vi "readMotorPodTurret.vi"(7 "Input Pod Clustor":T1, 8 "Pod Number":i32, 9 "Refnum in":T2) -> (1 "output cluster":T1)   [LabVIEW 2014]
uses:
  <vilib>/Utility/config.llb/Config Data RefNum.ctl
  read/readBooleanKey.vi
  read/readDoubleKey.vi
  read/readI32.vi
  read/readStringKey.vi
  <vilib>/Utility/config.llb/NI_LVConfig.lvlib
panel:
  in  "error in (no error)":errorcluster
  out "Refnum out":T2
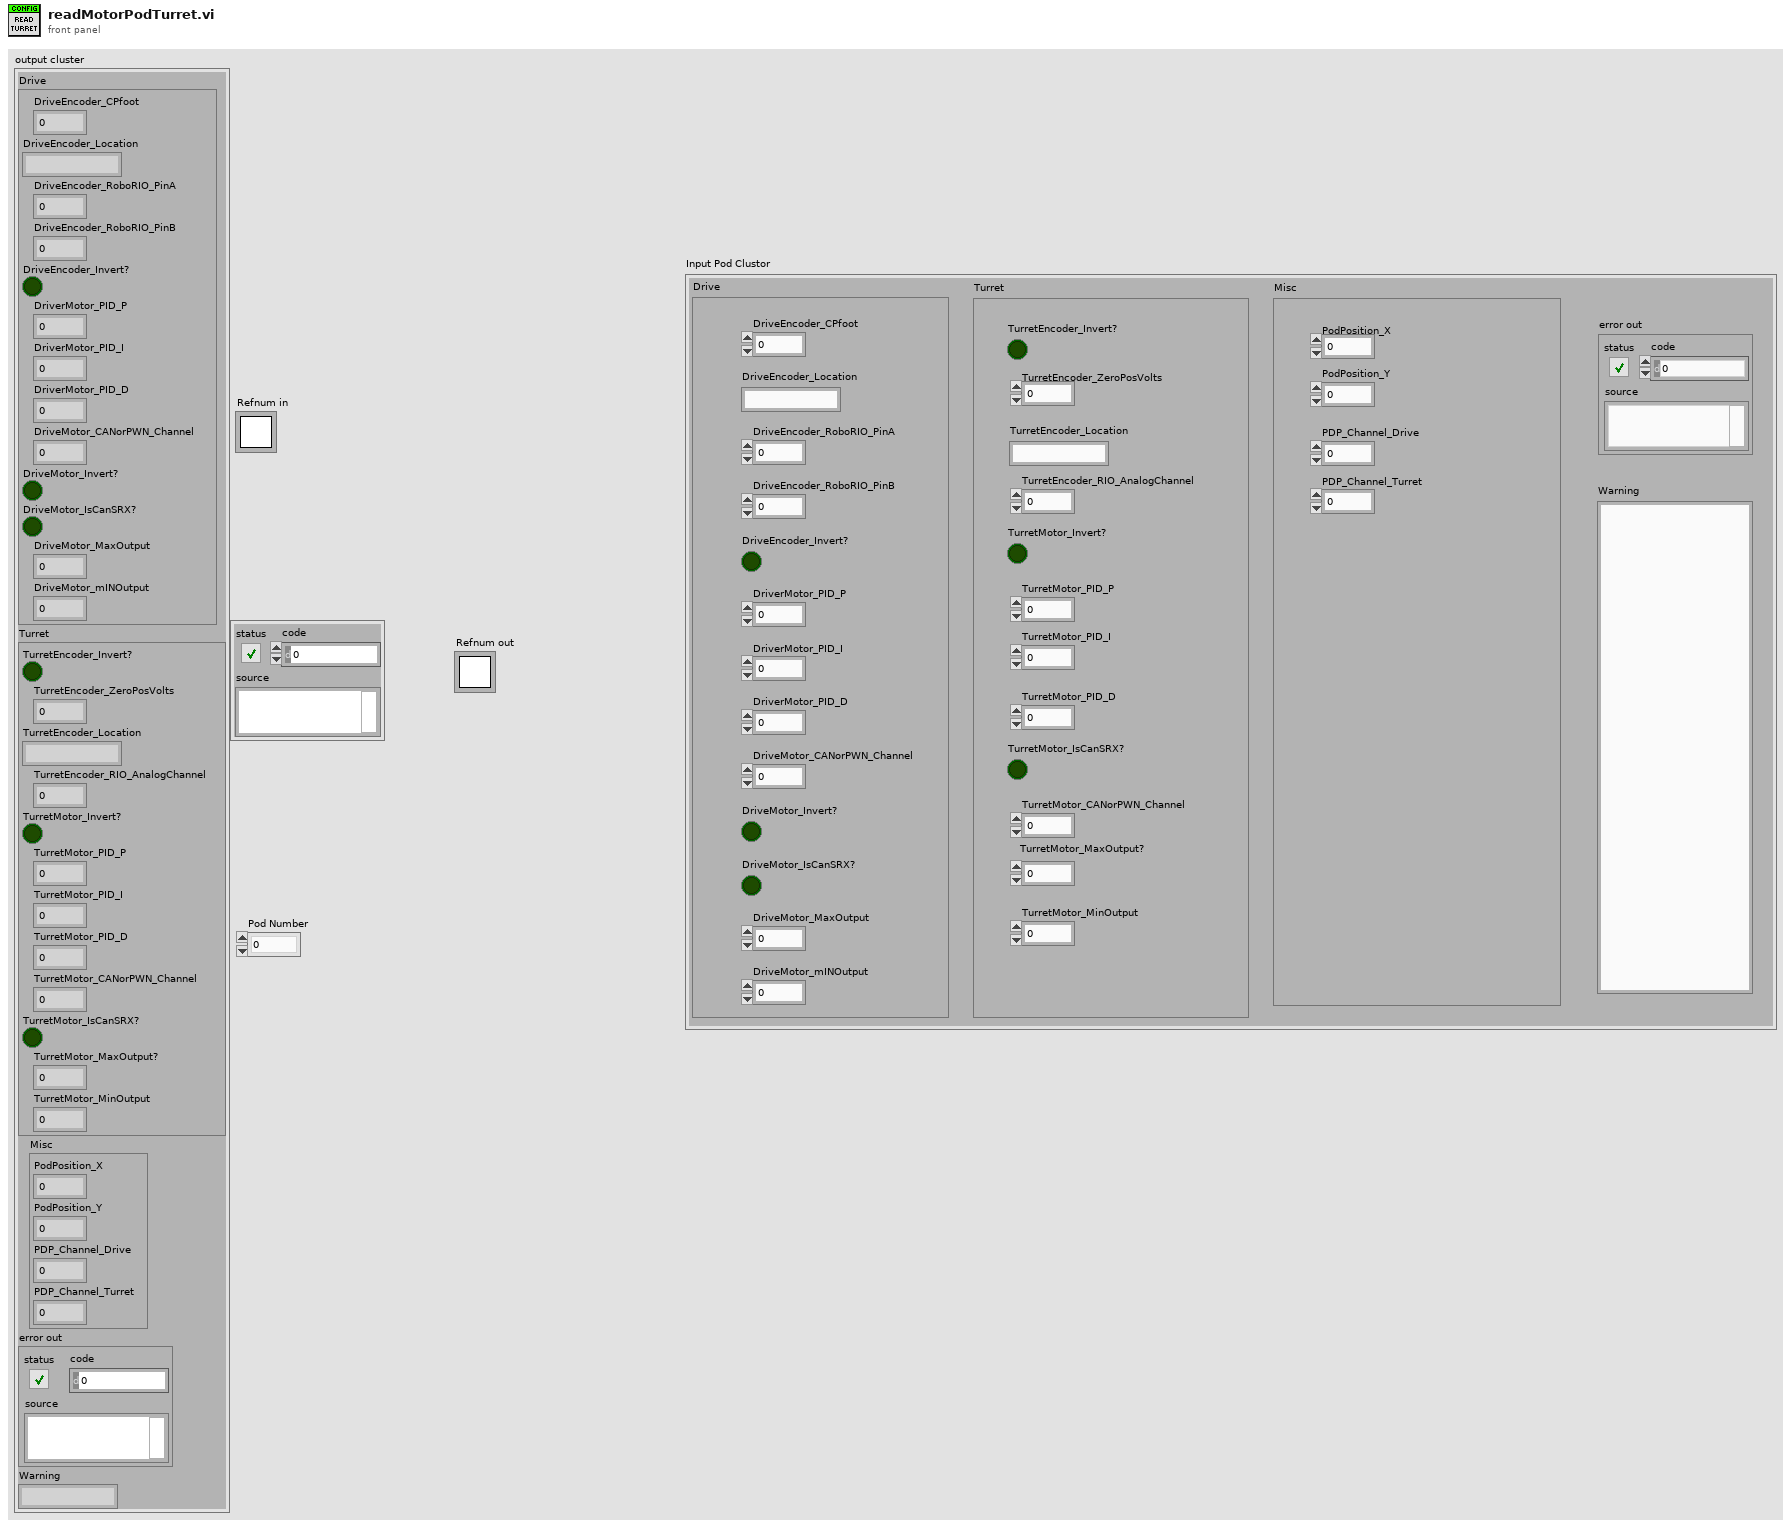
[diagram p1: front panel]
types:
  T1 = cluster{"Drive":cluster{"DriveEncoder_CPfoot":dbl, "DriveEncoder_Location":string, "DriveEncoder_RoboRIO_PinA":i32, "DriveEncoder_RoboRIO_PinB":i32, "DriveEncoder_Invert?":bool, "DriverMotor_PID_P":dbl, "DriverMotor_PID_I":dbl, "DriverMotor_PID_D":dbl, "DriveMotor_CANorPWN_Channel":i32, "DriveMotor_Invert?":bool, "DriveMotor_IsCanSRX?":bool, "DriveMotor_MaxOutput":dbl, "DriveMotor_mINOutput":dbl}, "Turret":cluster{"TurretEncoder_Invert?":bool, "TurretEncoder_ZeroPosVolts":dbl, "TurretEncoder_Location":string, "TurretEncoder_RIO_AnalogChannel":dbl, "TurretMotor_Invert?":bool, "TurretMotor_PID_P":dbl, "TurretMotor_PID_I":dbl, "TurretMotor_PID_D":dbl, "TurretMotor_CANorPWN_Channel":dbl, "TurretMotor_IsCanSRX?":bool, "TurretMotor_MaxOutput?":dbl, "TurretMotor_MinOutput":dbl}, "Misc":cluster{"PodPosition_X":dbl, "PodPosition_Y":dbl, "PDP_Channel_Drive":i32, "PDP_Channel_Turret":i32}, "error out":errorcluster, "Warning":string}
  T2 = typedef "NI_LVConfig.lvlib/Config Data RefNum.ctl" = refnum<k1>
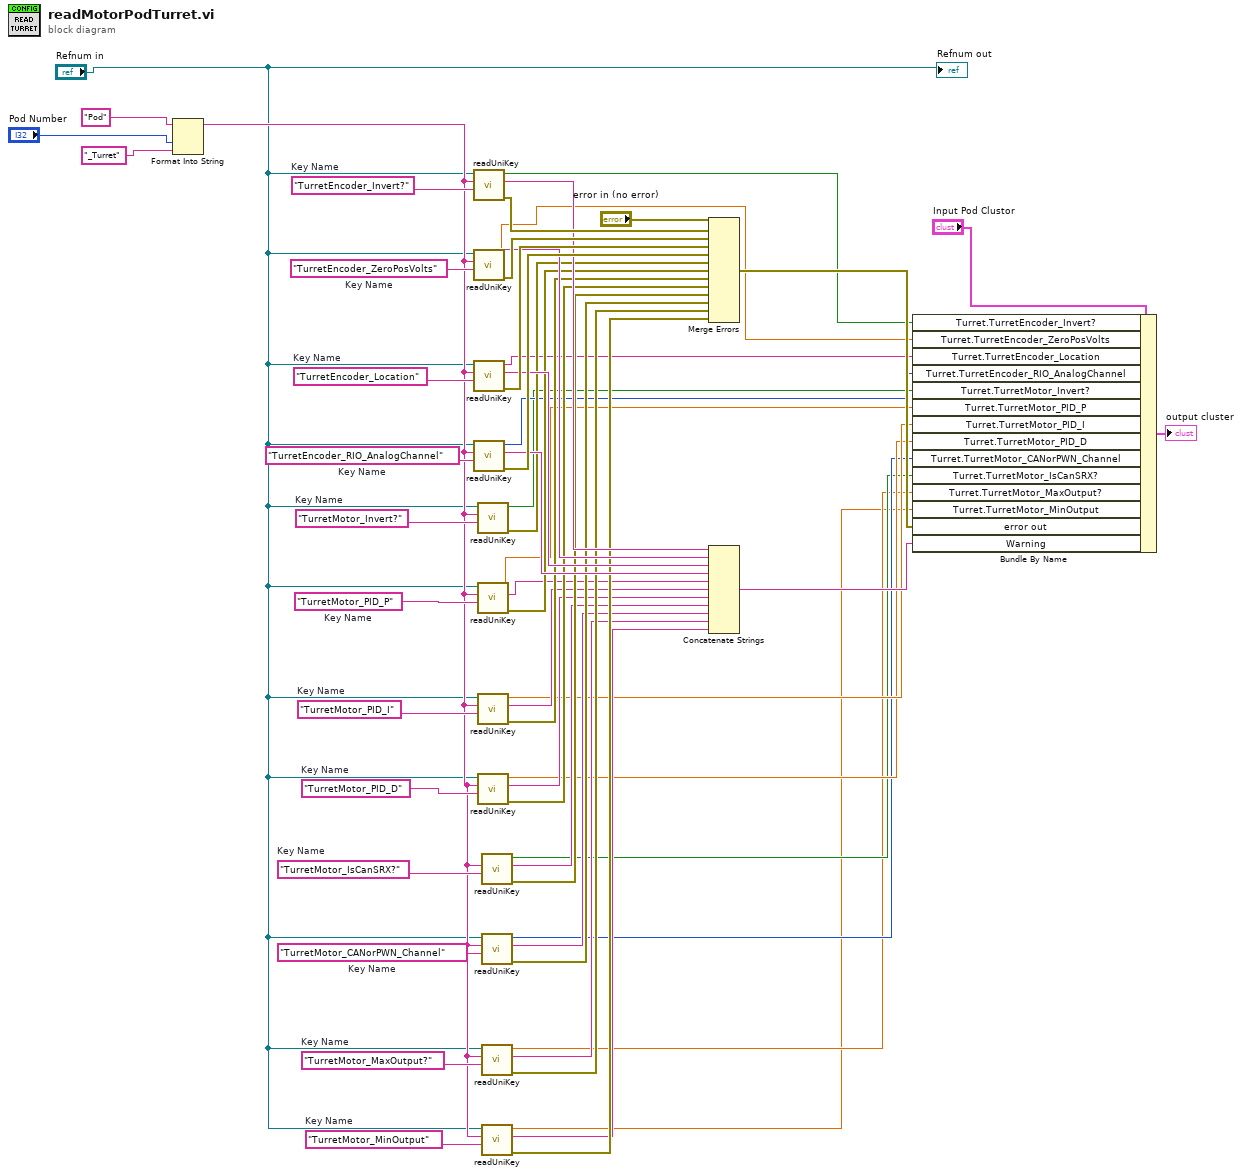
[diagram p0: block diagram]
diagram:
  w36 = "TurretMotor_MinOutput"  # Key Name
  w35 = "TurretMotor_MaxOutput?"  # Key Name
  w37 = "TurretMotor_CANorPWN_Channel"  # Key Name
  w38 = "TurretMotor_IsCanSRX?"  # Key Name
  w41 = "TurretMotor_PID_D"  # Key Name
  w42 = "TurretMotor_PID_I"  # Key Name
  w40 = "TurretMotor_PID_P"  # Key Name
  w39 = "TurretMotor_Invert?"  # Key Name
  w55 = "TurretEncoder_RIO_AnalogChannel"  # Key Name
  w54 = "TurretEncoder_Location"  # Key Name
  w56 = "TurretEncoder_ZeroPosVolts"  # Key Name
  w57 = "TurretEncoder_Invert?"  # Key Name
  n1 = Format Into String(initial string="Pod", "Pod Number", "_Turret") -> (resulting string=w34:string)  [unwired: 2 in, 1 out]
  n2 = call-poly "readUniKey.vi"("Refnum in"="Refnum in", "Section"=w34, "Key Name"=w57) -> ("value"=w13:bool, "Warning"=w49:string, "error out"=w53:errorcluster)  [unwired: 5 in]
  n3 = call-poly "readUniKey.vi"("Refnum in"="Refnum in", "Section"=w34, "Key Name"=w56) -> ("value"=w12:dbl, "Warning"=w48:string, "error out"=w52:errorcluster)  [unwired: 5 in]
  n4 = call-poly "readUniKey.vi"("Refnum in"="Refnum in", "Section"=w34, "Key Name"=w54) -> ("value"=w11:string, "Warning"=w47:string, "error out"=w51:errorcluster)  [unwired: 5 in]
  n5 = call-poly "readUniKey.vi"("Refnum in"="Refnum in", "Section"=w34, "Key Name"=w55) -> ("value"=w10:i32, "Warning"=w46:string, "error out"=w50:errorcluster)  [unwired: 5 in]
  n6 = call-poly "readUniKey.vi"("Refnum in"="Refnum in", "Section"=w34, "Key Name"=w39) -> ("value"=w9:bool, "error out"=w33:errorcluster)  [unwired: 5 in, 1 out]
  n7 = call-poly "readUniKey.vi"("Refnum in"="Refnum in", "Section"=w34, "Key Name"=w40) -> ("value"=w8:dbl, "Warning"=w25:string, "error out"=w32:errorcluster)  [unwired: 5 in]
  n8 = call-poly "readUniKey.vi"("Refnum in"="Refnum in", "Section"=w34, "Key Name"=w42) -> ("value"=w7:dbl, "Warning"=w24:string, "error out"=w31:errorcluster)  [unwired: 5 in]
  n9 = call-poly "readUniKey.vi"("Refnum in"="Refnum in", "Section"=w34, "Key Name"=w41) -> ("value"=w6:dbl, "Warning"=w23:string, "error out"=w30:errorcluster)  [unwired: 5 in]
  n10 = call-poly "readUniKey.vi"("Section"=w34, "Key Name"=w38) -> ("value"=w4:bool, "Warning"=w22:string, "error out"=w29:errorcluster)  [unwired: 6 in]
  n11 = call-poly "readUniKey.vi"("Refnum in"="Refnum in", "Section"=w34, "Key Name"=w37) -> ("value"=w5:i32, "Warning"=w21:string, "error out"=w28:errorcluster)  [unwired: 5 in]
  n12 = call-poly "readUniKey.vi"("Refnum in"="Refnum in", "Section"=w34, "Key Name"=w35) -> ("value"=w3:dbl, "Warning"=w20:string, "error out"=w27:errorcluster)  [unwired: 5 in]
  n13 = call-poly "readUniKey.vi"("Refnum in"="Refnum in", "Section"=w34, "Key Name"=w36) -> ("value"=w2:dbl, "Warning"=w19:string, "error out"=w26:errorcluster)  [unwired: 5 in]
  n14 = Merge Errors "Merge Errors"("error in (no error)", w53, w52, w51, w50, w33, w32, w31, w30, w29, w28, w27, w26) -> (w15:errorcluster)
  n15 = Concatenate Strings ("Concatenate Warnings")(w49, w48, w47, w46, w25, w24, w23, w22, w21, w20, w19) -> (w14:string)
  n16 = Bundle By Name(cluster="Input Pod Clustor", "Turret.TurretEncoder_Invert?"=w13, "Turret.TurretEncoder_ZeroPosVolts"=w12, "Turret.TurretEncoder_Location"=w11, "Turret.TurretEncoder_RIO_AnalogChannel"=w10, "Turret.TurretMotor_Invert?"=w9, "Turret.TurretMotor_PID_P"=w8, "Turret.TurretMotor_PID_I"=w7, "Turret.TurretMotor_PID_D"=w6, "Turret.TurretMotor_CANorPWN_Channel"=w5, "Turret.TurretMotor_IsCanSRX?"=w4, "Turret.TurretMotor_MaxOutput?"=w3, "Turret.TurretMotor_MinOutput"=w2, "error out"=w15, "Warning"=w14) -> (→"output cluster":T1)
  "Refnum out" <- "Refnum in"
